vi "Clear lines.vi"(0 "Section Y":i32, 5 "Section line":i32, 7 "Section X":i32, 9 "Section text":string, 11 "Display Array":string[][](array[string])) -> (4 "Stripped text":string, 15 "Cleared Display Array":string[][](array[string]))   [LabVIEW 2018]
uses:
  <vilib>/regexp/Match Regular Expression.xnode
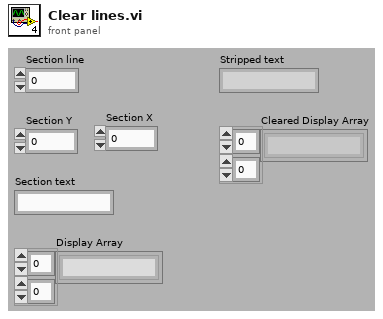
[diagram p1: front panel]
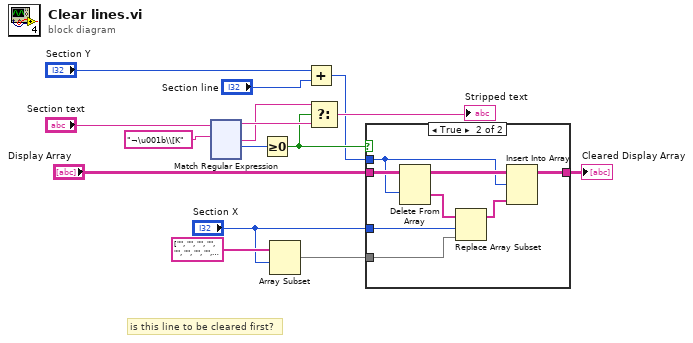
[diagram p0: block diagram]
diagram:
  # "is this line to be cleared first?"
  n1 = xnode "Match Regular Expression"("input string"="Section text", "regular expression"="¬\u001b\\[K" ("search string")) -> ("before match"=w14:string, "after match"=w13:string, "offset past match"=w5:i32)  [unwired: 4 in, 2 out]
  n2 = Greater Or Equal To 0?(x=w5) -> (x >= 0?=w12:bool)
  n3 = Array Subset(array=string[] ["", "", "", "", "", "", "", "", "", "", "", "", "", "", "", "", "", "", "", "", "", "", "", "", "", "", "", "", "", "", "", "", "", "", "", "", "", "", "", "", "", "", "", "", "", "", "", "", "", "", "", "", "", "", "", "", "", "", "", "", "", "", "", "", "", "", "", "", "", "", "", "", "", "", "", "", "", "", "", "", "", "", "", "", "", "", "", "", "", "", "", "", "", "", "", "", "", "", "", "", "", "", "", "", "", "", "", "", "", "", "", "", "", "", "", "", "", "", "", "", "", "", "", "", "", "", "", "", "", "", "", "", "", "", "", "", "", "", "", "", "", "", "", "", "", "", "", "", "", "", "", "", "", "", "", "", "", "", "", "", "", "", "", "", "", "", "", "", "", "", "", "", "", "", "", "", "", "", "", "", "", "", "", "", "", "", "", "", "", "", "", "", "", "", "", "", "", "", "", "", ""] ("Stripped Sections"), index="Section X") -> (w1:string[])  [unwired: 1 in]
  n4 = Add(x="Section Y", y="Section line") -> (x+y=w10:i32)
  n5 = Select(t=w13, s=w12, f=w14) -> (s? t:f=→"Stripped text":string)
  n6 = case shown="True" w12 {
    tunnel: "Display Array" -> [w16 w23]
    tunnel: [w16 w24] -> w9
    tunnel: w10 -> [_ w21]
    tunnel: "Section X" -> [_ w18]
    tunnel: w1 -> [_ w17]
    frame False {
    }
    frame True {
      n7 = Delete From Array(array=w23, index (row)=w21) -> (deleted portion=w20:string[], array with subset deleted=w22:string[][])  [unwired: 2 in]
      n8 = Replace Array Subset(array=w20, new element=w17, index=w18) -> (w19:string[])
      n9 = Insert Into Array(array=w22, index (row)=w21, new element=w19) -> (w24:string[][])  [unwired: 1 in]
    }
  }
  "Cleared Display Array" <- w9
